vi "PXDAC4800_GetSerialNumberXD48.vi"(0 "Handle":i32) -> (1 "Handle Out":i32, 2 "Status":i32, 3 "Serial num":i32)   [LabVIEW 2016]
uses:
  PXDAC4800.dll
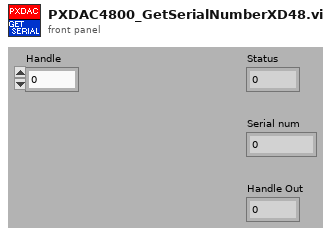
[diagram p1: front panel]
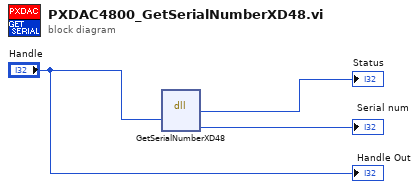
[diagram p0: block diagram]
diagram:
  n1 = dll-call lib="PXDAC4800.dll" fn="GetSerialNumberXD48"("Handle"="Handle") -> (→"Status":i32, "serial_num"=→"Serial num":u32)  [unwired: 5 in, 2 out]
  "Handle Out" <- "Handle"
